vi "Initialise All Aircraft Data.vi"(8 "Error In":errorcluster) -> (0 "Error Out":errorcluster)   [LabVIEW 2014]
uses:
  Controls/Drone Information.ctl
  Controls/Base Mode.ctl
  Controls/Aircraft Mode.ctl
  Telemetry/Controls/Telemetry Connection Type.ctl
  Controls/Aircraft RC Data.ctl
  Controls/Aircraft Attitude Data.ctl
  Set Aircraft Information.vi
  Set Aircraft RC.vi
  Set Aircraft Attitude.vi
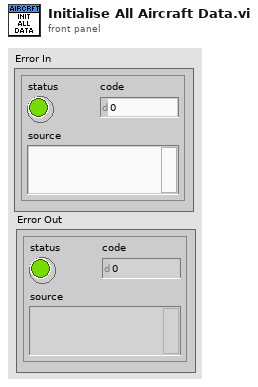
[diagram p1: front panel]
types:
  T1 = typedef "Aircraft Attitude Data.ctl" = cluster{"Roll":sgl, "Pitch":sgl, "Yaw":sgl, "Timestamp":u32, "Update Frequency":dbl, "Altitude":sgl}
  T2 = typedef "Aircraft RC Data.ctl" = cluster{"Channel 1 Min":i16, "Channel 1 Max":i16, "Channel 2 Min":i16, "Channel 2 Max":i16, "Channel 3 Min":i16, "Channel 3 Max":i16, "Channel 4 Min":i16, "Channel 4 Max":i16}
  T3 = typedef "Drone Information.ctl" = cluster{"Heart Beat":bool, "Aircraft ID":u8, "Downlink Port":refnum<visa-resource-name>, "Tag ID":string, "System Status":string, "Base Mode":T4, "Armed/Disarmed":bool, "Battery Voltage":dbl, "Control Mode":T5, "Initialisation":u8, "Heart Beat Status":bool, "Uplink Port":refnum<visa-resource-name>, "UDP connection ID":refnum<k16>, "Connection Type":T6, "Mode":string, "UDP IP Address":string, "Mission Uploaded":bool}
  T4 = typedef "Base Mode.ctl" = cluster{"Custom Mode":bool, "Test Enabled":bool, "Autonomous Mode":bool, "Guided Mode":bool, "Stabilization Enabled":bool, "HIL Enabled":bool, "Manual Mode":bool, "Arm":bool}
  T5 = typedef "Aircraft Mode.ctl" = enum16{"Loiter", "Stabalise", "Failsafe", "Emergency Stop"}
  T6 = typedef "Telemetry Connection Type.ctl" = enum16{"Serial", "UDP", "TCP"}
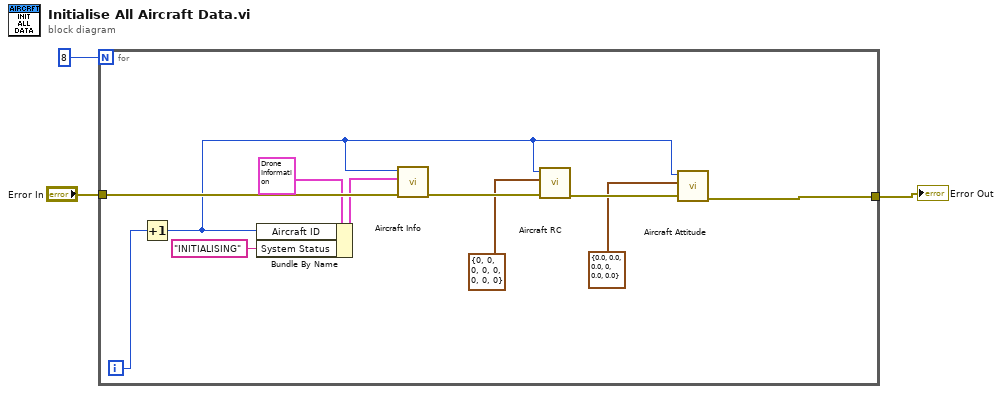
[diagram p0: block diagram]
diagram:
  n1 = for {
    N: 8 -> [_]
    tunnel: "Error In" -> [w14]
    tunnel: [w4] -> w1
    i -> [w7]
    n2 = Increment(x=w7) -> (x+1=w5:i32)
    n3 = Bundle By Name(cluster=T3 {"Heart Beat"=FALSE, "Aircraft ID"=0, "Downlink Port"="", "Tag ID"="", "System Status"="", "Base Mode"={"Custom Mode"=FALSE, "Test Enabled"=FALSE, "Autonomous Mode"=FALSE, "Guided Mode"=FALSE, "Stabilization Enabled"=FALSE, "HIL Enabled"=FALSE, "Manual Mode"=FALSE, "Arm"=FALSE}, "Armed/Disarmed"=FALSE, "Battery Voltage"=0.0, "Control Mode"=enum."Stabalise", "Initialisation"=0, "Heart Beat Status"=FALSE, "Uplink Port"="", "UDP connection ID"=refnum, "Connection Type"=enum."Serial", "Mode"="", "UDP IP Address"="", "Mission Uploaded"=FALSE} ("Aircraft Information In"), "Aircraft ID"=w5, "System Status"="INITIALISING") -> (w8:T3)
    n4 = call-poly "Aircraft Info.vi"("Error In"=w14, "Aircraft Information In"=w8, "Aircraft ID"=w5) -> ("Error Out"=w13:errorcluster)  [unwired: 8 in]
    n5 = call-poly "Aircraft RC.vi"("Error In"=w13, "Aircraft RC Data"=T2 {"Channel 1 Min"=0, "Channel 1 Max"=0, "Channel 2 Min"=0, "Channel 2 Max"=0, "Channel 3 Min"=0, "Channel 3 Max"=0, "Channel 4 Min"=0, "Channel 4 Max"=0}, "Aircraft ID"=w5) -> ("Error Out"=w12:errorcluster)  [unwired: 8 in]
    n6 = call-poly "Aircraft Attitude.vi"("Error In"=w12, "Aircraft Att Data"=T1 {"Roll"=0.0, "Pitch"=0.0, "Yaw"=0.0, "Timestamp"=0, "Update Frequency"=0.0, "Altitude"=0.0}, "Aircraft ID"=w5) -> ("Error Out"=w4:errorcluster)  [unwired: 8 in]
  }
  "Error Out" <- w1
